vi "Choose Color Table.vi"(8 "Size (256)":i32=256, 9 "Custom Table":u32[](array[colorbox])=[0, 4718676, 5189759, 4414349, 3440526, 2269831, 4047724, 9689909, 15984924, 10420479, 16860, 3381759, 6618880, 16772608, 16711680], 10 "ColorCET":T2(ring), 11 "Color Map":T1(ring)=enum."Viridis") -> (0 "B []":u8[](array[numeric])=[0, 5, 9, 14, 18, 23, 28, 32, 37, 42, 46, 51, 55, 60, 65, 69, 74, 78, 83, 86, 88, 91, 93, 95, 98, 100, 102, 105, 107, 109, 112, 114, 117, 119, 121, 124, 126, 127, 128, 129, 130, 131, 131, 132, 133, 134, 134, 135, 136, 137, 137, 138, 139, 140, 141, 141, 141, 141, 141, 141, 141, 141, 141, 141, 142, 142, 142, 142, 142, 142, 142, 142, 142, 142, 142, 141, 141, 140, 140, 140, 139, 139, 138, 138, 138, 137, 137, 137, 136, 136, 135, 135, 134, 132, 131, 129, 128, 126, 125, 123, 122, 120, 119, 117, 116, 114, 113, 111, 110, 108, 106, 103, 100, 97, 94, 91, 88, 85, 82, 79, 76, 73, 70, 67, 64, 61, 58, 55, 52, 51, 50, 48, 47, 45, 44, 43, 41, 40, 39, 37, 36, 34, 33, 32, 30, 29, 32, 44, 56, 69, 81, 94, 106, 119, 131, 144, 156, 169, 181, 194, 206, 219, 231, 243, 255, 253, 251, 249, 247, 245, 243, 241, 239, 238, 236, 234, 232, 230, 228, 226, 224, 222, 220, 222, 224, 225, 227, 229, 231, 233, 235, 237, 239, 241, 243, 245, 247, 249, 250, 252, 254, 246, 232, 218, 204, 190, 176, 162, 148, 134, 120, 106, 92, 78, 64, 50, 36, 22, 8, 0, 0, 0, 0, 0, 0, 0, 0, 0, 0, 0, 0, 0, 0, 0, 0, 0, 0, 0, 0, 0, 0, 0, 0, 0, 0, 0, 0, 0, 0, 0, 0, 0, 0, 0, 0, 0], 1 "G []":u8[](array[numeric])=[0, 0, 0, 0, 0, 0, 0, 0, 0, 0, 0, 0, 0, 0, 0, 0, 0, 0, 0, 2, 5, 7, 10, 13, 15, 18, 21, 23, 26, 28, 31, 34, 36, 39, 42, 44, 47, 49, 52, 54, 56, 59, 61, 64, 66, 68, 71, 73, 75, 78, 80, 82, 85, 87, 89, 92, 94, 96, 98, 100, 102, 104, 106, 108, 109, 111, 113, 115, 117, 119, 121, 123, 125, 127, 129, 131, 133, 135, 137, 139, 141, 143, 145, 146, 148, 150, 152, 154, 156, 158, 160, 162, 164, 165, 167, 169, 171, 173, 175, 176, 178, 180, 182, 184, 185, 187, 189, 191, 193, 194, 196, 197, 199, 200, 201, 203, 204, 205, 206, 208, 209, 210, 212, 213, 214, 216, 217, 218, 219, 220, 221, 222, 222, 223, 224, 225, 226, 226, 227, 228, 229, 229, 230, 231, 232, 232, 229, 217, 204, 191, 178, 165, 153, 140, 127, 114, 101, 89, 76, 63, 50, 37, 25, 12, 0, 4, 7, 11, 15, 18, 22, 25, 29, 32, 36, 40, 43, 47, 50, 54, 57, 61, 64, 69, 74, 79, 84, 88, 93, 98, 103, 108, 113, 117, 122, 127, 132, 137, 142, 146, 151, 157, 162, 168, 173, 179, 185, 190, 196, 201, 207, 213, 218, 224, 229, 235, 241, 246, 252, 255, 254, 253, 252, 251, 250, 249, 248, 247, 246, 245, 244, 243, 242, 242, 241, 240, 239, 235, 222, 209, 196, 183, 170, 157, 144, 131, 118, 105, 91, 78, 65, 52, 39, 26, 13, 0], 2 "R []":u8[](array[numeric])=[0, 4, 8, 12, 16, 20, 24, 28, 32, 36, 40, 43, 47, 51, 55, 59, 63, 67, 71, 72, 73, 73, 73, 74, 74, 75, 75, 75, 76, 76, 77, 77, 77, 78, 78, 78, 79, 79, 78, 77, 77, 76, 75, 75, 74, 73, 73, 72, 71, 71, 70, 69, 69, 68, 67, 67, 66, 65, 64, 63, 63, 62, 61, 60, 59, 58, 58, 57, 56, 55, 54, 54, 53, 52, 51, 50, 49, 48, 47, 46, 45, 44, 43, 42, 41, 40, 39, 38, 37, 36, 35, 34, 35, 37, 38, 40, 41, 43, 44, 46, 47, 49, 50, 52, 53, 55, 56, 58, 59, 61, 64, 69, 74, 79, 83, 88, 93, 97, 102, 107, 112, 116, 121, 126, 130, 135, 140, 145, 150, 155, 160, 165, 171, 176, 181, 187, 192, 197, 202, 208, 213, 218, 223, 229, 234, 239, 242, 237, 232, 228, 223, 219, 214, 209, 205, 200, 196, 191, 186, 182, 177, 173, 168, 163, 158, 150, 141, 132, 123, 115, 106, 97, 89, 80, 71, 62, 54, 45, 36, 27, 19, 10, 1, 2, 5, 8, 11, 14, 16, 19, 22, 25, 28, 30, 33, 36, 39, 42, 44, 47, 50, 53, 55, 58, 61, 63, 66, 69, 72, 74, 77, 80, 82, 85, 88, 90, 93, 96, 98, 104, 112, 121, 129, 138, 146, 155, 163, 172, 180, 189, 197, 206, 214, 223, 231, 240, 248, 255, 255, 255, 255, 255, 255, 255, 255, 255, 255, 255, 255, 255, 255, 255, 255, 255, 255, 255], 3 "Color Table":u32[](array[colorbox])=[0, 262149, 524297, 786446, 1048594, 1310743, 1572892, 1835040, 2097189, 2359338, 2621486, 2818099, 3080247, 3342396, 3604545, 3866693, 4128842, 4390990, 4653139, 4719190, 4785496, 4786011, 4786781, 4853087, 4853602, 4919908, 4920678, 4921193, 4987499, 4988013, 5054320, 5055090, 5055605, 5121911, 5122681, 5123196, 5189502, 5190015, 5125248, 5060225, 5060738, 4995971, 4930947, 4931716, 4866693, 4801670, 4802438, 4737415, 4672392, 4673161, 4608137, 4543114, 4543883, 4478860, 4413837, 4414605, 4349581, 4284557, 4219533, 4154509, 4155021, 4089997, 4024973, 3959949, 3894670, 3829646, 3830158, 3765134, 3700110, 3635086, 3570062, 3570574, 3505550, 3440526, 3375502, 3310477, 3245453, 3180428, 3115404, 3050380, 2985355, 2920331, 2855306, 2790026, 2725002, 2659977, 2594953, 2529929, 2464904, 2399880, 2334855, 2269831, 2335878, 2467204, 2533251, 2664833, 2730880, 2862462, 2928509, 3059835, 3125882, 3257464, 3323511, 3455093, 3520884, 3652466, 3718513, 3850095, 3916142, 4047468, 4244586, 4572519, 4900708, 5228641, 5491038, 5819227, 6147160, 6409557, 6737490, 7065679, 7393612, 7656009, 7984198, 8312131, 8574528, 8902717, 9230650, 9558583, 9886516, 10214451, 10542386, 10870320, 11263535, 11591469, 11919404, 12312875, 12640809, 12968488, 13296423, 13689893, 14017828, 14345506, 14673441, 15066912, 15394846, 15722525, 15918368, 15587628, 15256632, 14991173, 14660177, 14394718, 14063978, 13732983, 13467523, 13136528, 12871068, 12540329, 12209333, 11943874, 11612878, 11347419, 11016679, 10685683, 10354943, 9831677, 9242619, 8653817, 8065015, 7541493, 6952691, 6363633, 5840367, 5251310, 4662508, 4073706, 3550184, 2961382, 2372324, 1783522, 1260000, 671198, 82140, 148958, 346848, 544737, 742627, 940261, 1072615, 1270505, 1468395, 1666285, 1864175, 1996273, 2194163, 2392053, 2589943, 2787833, 2920186, 3117820, 3315710, 3513846, 3646184, 3844314, 4042188, 4174782, 4372912, 4570786, 4768916, 4901254, 5099384, 5297514, 5429852, 5627982, 5825856, 5958450, 6156580, 6354454, 6487048, 6881024, 7405056, 7994624, 8518656, 9108224, 9632256, 10221824, 10745856, 11335424, 11859456, 12449024, 12973056, 13562624, 14086656, 14676480, 15200512, 15790080, 16314112, 16771840, 16768512, 16765184, 16761856, 16758528, 16755200, 16751872, 16748544, 16745216, 16741888, 16738560, 16734976, 16731648, 16728320, 16724992, 16721664, 16718336, 16715008, 16711680])   [LabVIEW 2019, in "graph_utilities.lvclass"]
doc: "Choose a color table for your graph by name\n<b>Color Table</b>:\n- Inferno\n- Kindlmann\n- Plasma\n- Viritis [Default]\n- LevyLab2010 (Rainbow)\n- ColorCET: Perceptually Uniform Color Maps\n - Choose with <b>ColorCET</b> control\n- Custom:\n - Choose with <b>Custom Table</b> control\n\n<b>Size</b>Choose number of colors in output table."
uses:
  graph_utilities.lvclass
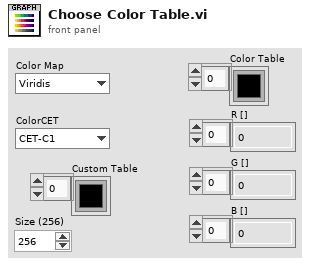
[diagram p1: front panel]
types:
  T1 = enum16{"Inferno", "Kindlmann", "Plasma", "Viridis", "LevyLab2010", "ColorCET...", "Custom..."}
  T2 = enum16{"CET-C1", "CET-C1s", "CET-C2", "CET-C2s", "CET-C3", "CET-C3s", "CET-C4", "CET-C4s", "CET-C5", "CET-C5s", "CET-C6", "CET-C6s", "CET-C7", "CET-C7s", "CET-CBC1", "CET-CBC2", "CET-CBD1", "CET-CBL1", "CET-CBL2", "CET-D01", "CET-D01A", "CET-D02", "CET-D03", "CET-D04", "CET-D06", "CET-D07", "CET-D08", "CET-D09", "CET-D10", "CET-D11", "CET-D12", "CET-D13", "CET-I1", "CET-I2", "CET-I3", "CET-L01", "CET-L02", "CET-L03", "CET-L04", "CET-L05", "CET-L06", "CET-L07", "CET-L08", "CET-L09", "CET-L10", "CET-L11", "CET-L12", "CET-L13", "CET-L14", "CET-L15", "CET-L16", "CET-L17", "CET-L18", "CET-L19", "CET-L20", "CET-R1", "CET-R2", "CET-R3", "CET-R4"}
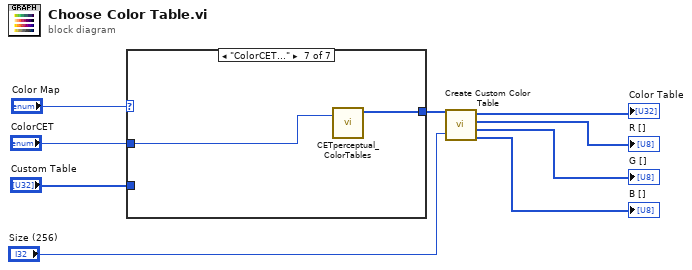
[diagram p0: block diagram]
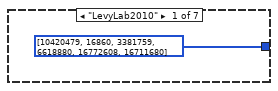
[diagram p2: hidden frame]
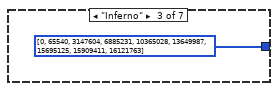
[diagram p4: hidden frame]
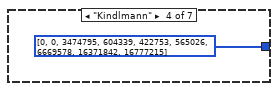
[diagram p5: hidden frame]
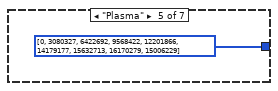
[diagram p6: hidden frame]
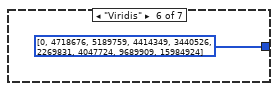
[diagram p7: hidden frame]
diagram:
  n1 = case shown="\"ColorCET...\"" "Color Map" {
    tunnel: [u32[] [10420479, 16860, 3381759, 6618880, 16772608, 16711680] ("Colors []") w11 u32[] [0, 65540, 3147604, 6885231, 10365028, 13649987, 15695125, 15909411, 16121763] ("Colors []") u32[] [0, 0, 3474795, 604339, 422753, 565026, 6669578, 16371842, 16777215] ("Colors []") u32[] [0, 3080327, 6422692, 9568422, 12201866, 14179177, 15632713, 16170279, 15006229] ("Colors []") u32[] [0, 4718676, 5189759, 4414349, 3440526, 2269831, 4047724, 9689909, 15984924] ("Colors []") w17] -> w6
    tunnel: "ColorCET" -> [_ _ _ _ _ _ w16]
    tunnel: "Custom Table" -> [_ w11 _ _ _ _ _]
    frame "LevyLab2010" {
    }
    frame "Custom..." {
    }
    frame "Inferno" {
    }
    frame "Kindlmann" {
    }
    frame "Plasma" {
    }
    frame "Viridis" {
    }
    frame "ColorCET..." {
      n2 = call "CETperceptual_ColorTables.vi"("CET"=w16) -> ("Color Table"=w17:u32[])  [unwired: 1 in, 3 out]
    }
  }
  n3 = call "Create Custom Color Table.vi"("Colors []"=w6, "Size (256)"="Size (256)") -> ("Color Tbl"=→"Color Table":u32[], "R []"=→"R []":u8[], "G []"=→"G []":u8[], "B []"=→"B []":u8[])
